vi "uTTA_SetAnalogSettings.vi"(4 "Calibration Mode":bool, 5 "error in":errorcluster, 6 "Set Value":dbl, 7 "Channel":enum16{"ISEN", "SPARE", "VOFF0", "VOFF1"}(ring), 8 "VISA Refnum in":refnum<visa-resource-name>) -> (0 "error out":errorcluster, 1 "Received":string, 3 "VISA Refnum out":refnum<visa-resource-name>)   [LabVIEW 2021]
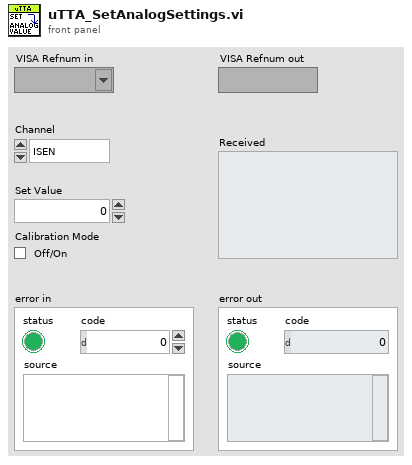
[diagram p1: front panel]
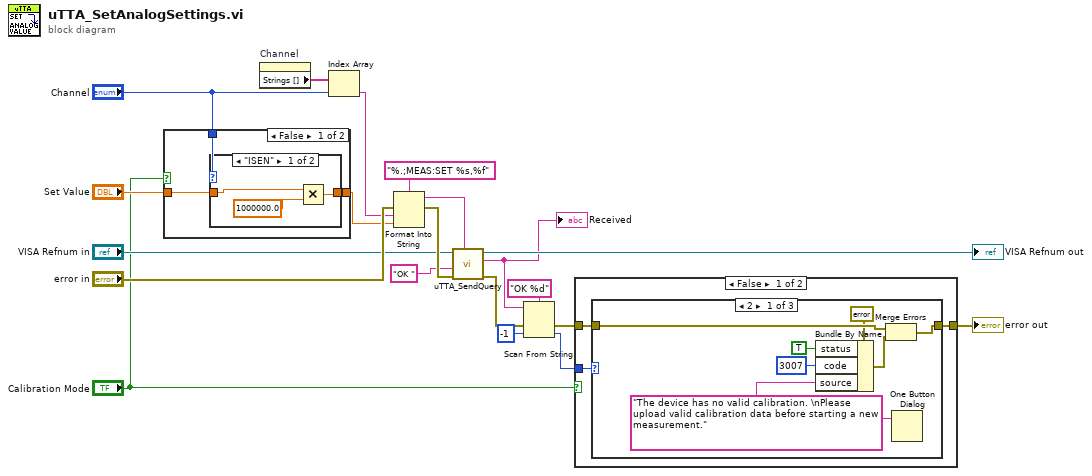
[diagram p0: block diagram]
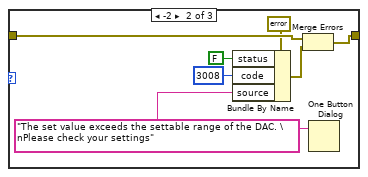
[diagram p2: hidden frame]
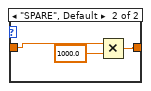
[diagram p5: hidden frame]
diagram:
  n1 = case shown="False" "Calibration Mode" {
    tunnel: "Channel" -> [w23 _]
    tunnel: "Set Value" -> [w22 w30]
    tunnel: [w21 w30] -> w11
    frame False {
      n2 = case shown="\"ISEN\"" w23 {
        tunnel: w22 -> [w25 w29]
        tunnel: [w26 w28] -> w21
        frame "ISEN" {
          n3 = Multiply(x=w25, y=1000000.0) -> (x*y=w26:dbl)
        }
        frame "SPARE", Default {
          n4 = Multiply(x=w29, y=1000.0) -> (x*y=w28:dbl)
        }
      }
    }
    frame True {
    }
  }
  n5 = property on="Channel" class="Enum (strict)"() -> ("Strings []"=w15:string[])  [unwired: 2 in, 2 out]
  n6 = Index Array(array=w15, index="Channel") -> (element=w14:string)
  n7 = Format Into String(format string="%.;MEAS:SET %s,%f", error in="error in", w14, w11) -> (resulting string=w10:string, error out=w20:errorcluster)  [unwired: 1 in]
  n8 = call "uTTA_SendQuery.vi"("Send String"=w10, "error in (no error)"=w20, "Response Qualifier(\"\")"="OK " ("Response Qualifier(\"\")"), "VISA Refnum in"="VISA Refnum in") -> ("error out"=w1:errorcluster, "Received"=w9:string, "VISA Refnum out"=→"VISA Refnum out":refnum<visa-resource-name>)  [unwired: 5 in]
  "Received" <- w9
  n9 = Scan From String(format string="OK %d", input string=w9, error in=w1, default 1=-1 ("default value 1")) -> (error out=w5:errorcluster, output 1=w7:i32)  [unwired: 1 in, 2 out]
  n10 = case shown="False" "Calibration Mode" {
    tunnel: w7 -> [w33 _]
    tunnel: w5 -> [w32 w49]
    tunnel: [w31 w49] -> w4
    frame False {
      n11 = case shown="2" w33 {
        tunnel: w32 -> [w40 w47 w48]
        tunnel: [w39 w46 w48] -> w31
        frame 2 {
          w34 = "The device has no valid calibration. \nPlease upload valid calibration data before starting a new measurement." ("message")
          n12 = Bundle By Name(cluster=errorcluster {"status"=FALSE, "code"=0, "source"=""} ("error in"), "status"=TRUE, "code"=3007, "source"=w34) -> (w37:errorcluster)
          n13 = Merge Errors(w40, w37) -> (w39:errorcluster)
          n14 = One Button Dialog(message=w34) -> ()  [unwired: 1 in, 1 out]
        }
        frame -2 {
          w41 = "The set value exceeds the settable range of the DAC. \nPlease check your settings" ("message")
          n15 = Bundle By Name(cluster=errorcluster {"status"=FALSE, "code"=0, "source"=""} ("error in"), "status"=FALSE, "code"=3008, "source"=w41) -> (w44:errorcluster)
          n16 = Merge Errors(w47, w44) -> (w46:errorcluster)
          n17 = One Button Dialog(message=w41) -> ()  [unwired: 1 in, 1 out]
        }
        frame 1, Default {
        }
      }
    }
    frame True {
    }
  }
  "error out" <- w4
